vi "Enqueue Message Poly.vi"   [LabVIEW 2023, in "Message Queue.lvlib"]
uses:
  Message Queue.lvlib
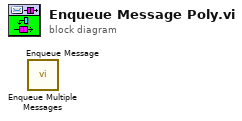
[diagram p0: block diagram]
diagram:
  n1 = call "Enqueue Multiple Messages.vi"() -> ()  [unwired: 11 in, 1 out]
  n2 = call "Enqueue Message.vi"() -> ()  [unwired: 11 in, 1 out]
